vi "GetInputQtyM100.vi"(8 "error in (no error)":errorcluster, 9 "Step":string, 10 "RCNO":string, 11 "connection reference":T1) -> (0 "error out":errorcluster, 2 "InputQty":i32, 3 "connection reference 2":T1)   [LabVIEW 2012]
uses:
  <vilib>/addons/database/Connection.llb/Conn ObjectReference.ctl
  <vilib>/addons/database/Auxilliary.llb/DB Tools Cursor Type.ctl
  <vilib>/addons/database/Connection.llb/Conn Execute.vi
  <vilib>/addons/database/Recordset.llb/Rec Fetch Integer Data (R).vi
  <vilib>/addons/database/Recordset.llb/Rec Destroy - Connection.vi
  <vilib>/addons/database/NI_Database_API.lvlib
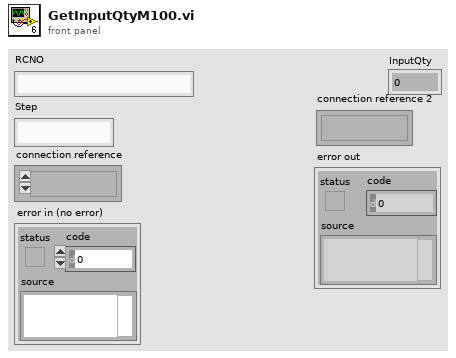
[diagram p1: front panel]
types:
  T1 = typedef "NI_Database_API.lvlib/Conn ObjectReference.ctl" = refnum<k1>
  T2 = typedef "NI_Database_API.lvlib/DB Tools Cursor Type.ctl" = enum16{"forward-only", "keyset", "dynamic", "static"}
  T3 = typedef "NI_Database_API.lvlib/Rec ObjectReference.ctl" = refnum<k1>
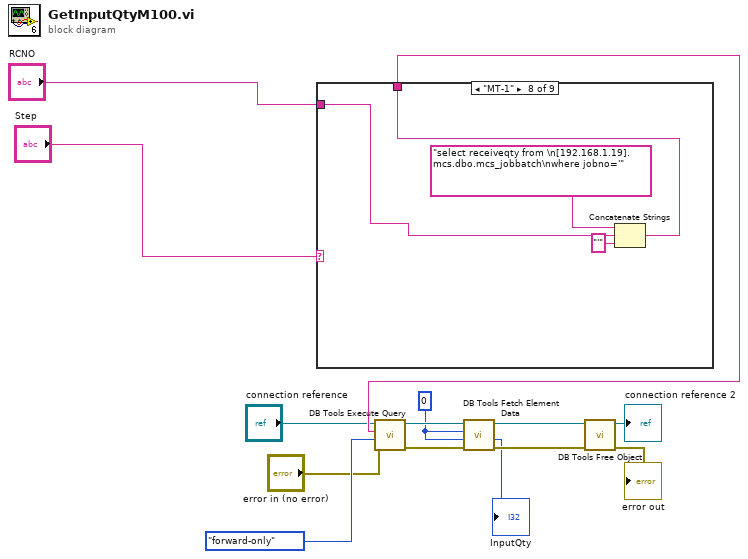
[diagram p0: block diagram]
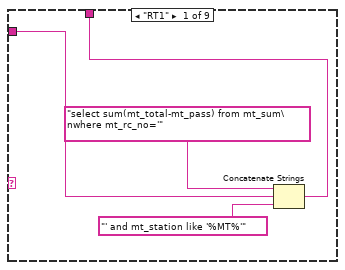
[diagram p2: hidden frame]
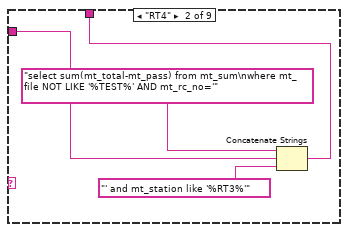
[diagram p3: hidden frame]
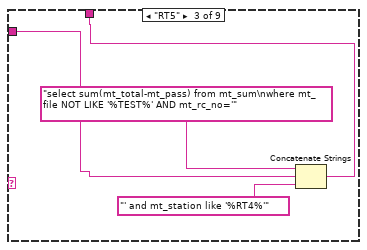
[diagram p4: hidden frame]
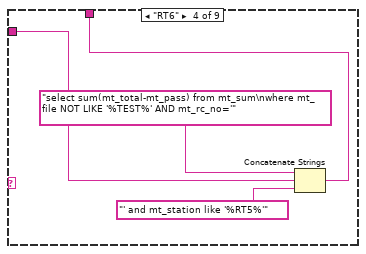
[diagram p5: hidden frame]
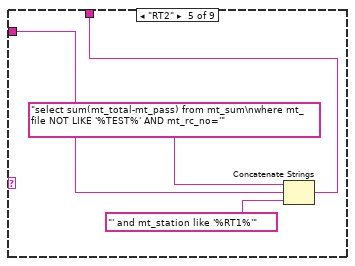
[diagram p6: hidden frame]
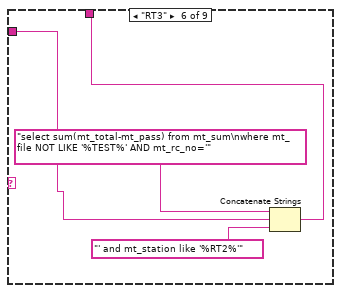
[diagram p7: hidden frame]
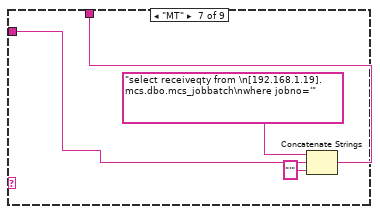
[diagram p8: hidden frame]
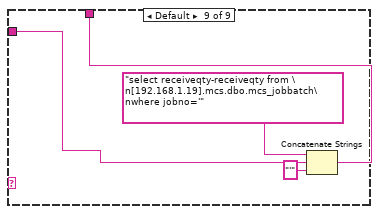
[diagram p9: hidden frame]
diagram:
  w6 = 0
  n1 = case shown="\"MT-1\"" "Step" {
    tunnel: "RCNO" -> [w16 w19 w24 w27 w32 w35 w41 w45 w49]
    tunnel: [w15 w20 w23 w28 w31 w36 w40 w44 w48] -> w7
    frame "RT1" {
      n2 = Concatenate Strings("select sum(mt_total-mt_pass) from mt_sum\nwhere mt_rc_no='" ("string"), w16, "' and mt_station like '%MT%'" ("string")) -> (w15:string)
    }
    frame "RT4" {
      n3 = Concatenate Strings("select sum(mt_total-mt_pass) from mt_sum\nwhere mt_file NOT LIKE '%TEST%' AND mt_rc_no='" ("string"), w19, "' and mt_station like '%RT3%'" ("string")) -> (w20:string)
    }
    frame "RT5" {
      n4 = Concatenate Strings("select sum(mt_total-mt_pass) from mt_sum\nwhere mt_file NOT LIKE '%TEST%' AND mt_rc_no='" ("string"), w24, "' and mt_station like '%RT4%'" ("string")) -> (w23:string)
    }
    frame "RT6" {
      n5 = Concatenate Strings("select sum(mt_total-mt_pass) from mt_sum\nwhere mt_file NOT LIKE '%TEST%' AND mt_rc_no='" ("string"), w27, "' and mt_station like '%RT5%'" ("string")) -> (w28:string)
    }
    frame "RT2" {
      n6 = Concatenate Strings("select sum(mt_total-mt_pass) from mt_sum\nwhere mt_file NOT LIKE '%TEST%' AND mt_rc_no='" ("string"), w32, "' and mt_station like '%RT1%'" ("string")) -> (w31:string)
    }
    frame "RT3" {
      n7 = Concatenate Strings("select sum(mt_total-mt_pass) from mt_sum\nwhere mt_file NOT LIKE '%TEST%' AND mt_rc_no='" ("string"), w35, "' and mt_station like '%RT2%'" ("string")) -> (w36:string)
    }
    frame "MT" {
      n8 = Concatenate Strings("select receiveqty from \n[192.168.1.19].mcs.dbo.mcs_jobbatch\nwhere jobno='" ("string"), w41, "'" ("string")) -> (w40:string)
    }
    frame "MT-1" {
      n9 = Concatenate Strings("select receiveqty from \n[192.168.1.19].mcs.dbo.mcs_jobbatch\nwhere jobno='" ("string"), w45, "'" ("string")) -> (w44:string)
    }
    frame Default {
      n10 = Concatenate Strings("select receiveqty-receiveqty from \n[192.168.1.19].mcs.dbo.mcs_jobbatch\nwhere jobno='" ("string"), w49, "'" ("string")) -> (w48:string)
    }
  }
  n11 = call-poly <vilib>:"DB Tools Execute Query.vi"("error in (no error)"="error in (no error)", "cursor type"=DB_Tools_Cursor_Type."forward-only", "SQL query"=w7, "connection reference"="connection reference") -> ("error out"=w13:errorcluster, "recordset reference"=w14:T3)  [unwired: 4 in]
  n12 = call-poly <vilib>:"DB Tools Fetch Element Data.vi"("error in (no error)"=w13, "type"=w6, "column index"=w6, "recordset reference"=w14) -> ("error out"=w11:errorcluster, "data"=→"InputQty":i32, "recordset reference out"=w12:T3)  [unwired: 3 in]
  n13 = call-poly <vilib>:"DB Tools Free Object.vi"("error in (no error)"=w11, "recordset reference"=w12) -> ("error out"=→"error out":errorcluster, "connection reference"=→"connection reference 2":T1)  [unwired: 8 in]
